vi "Set Config Ref.vi"(8 "error in (no error)":errorcluster, 10 "Reference":variant, 11 "Configuration In":refnum<class "Configuration.lvclass">) -> (0 "error out":errorcluster, 3 "Configuration Out":refnum<class "Configuration.lvclass">)   [LabVIEW 2020, in "Configuration.lvclass"]
doc: "For the configuration interface to work, the class implementing the interface needs to save the reference to the implementation in the class attributes. This is an accessor for that attribute which must be implemented by the class."
uses:
  Configuration.lvclass
  Base/Base.lvclass
  Base/Base.lvclass/Base.ctl
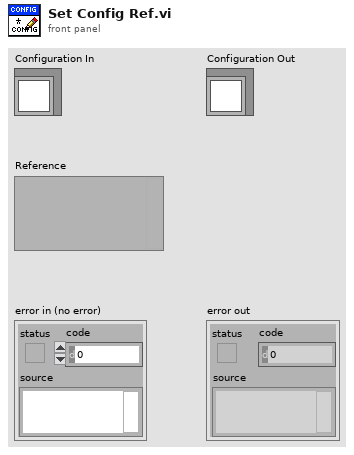
[diagram p1: front panel]
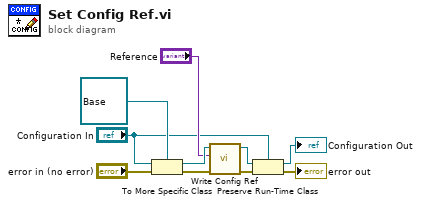
[diagram p0: block diagram]
diagram:
  n1 = To More Specific Class(target class=refnum<class "Base.lvclass"> refnum ("Base.lvclass"), reference="Configuration In", error in="error in (no error)") -> (specific class reference=w9:refnum<class "Base.lvclass">, error out=w8:errorcluster)
  n2 = call "Write Config Ref.vi"("error in (no error)"=w8, "Config File Refnum"="Reference", "Base In"=w9) -> ("error out"=w5:errorcluster, "Base Out"=w3:refnum<class "Base.lvclass">)  [unwired: 7 in]
  n3 = Preserve Run-Time Class(object in=w3, error in=w5, 2:"Configuration In") -> (object out=→"Configuration Out":refnum<class "Configuration.lvclass">, error out=→"error out":errorcluster)
